vi "PlotCylDBparams.vi"() -> ()   [LabVIEW 2014]
uses:
  TypeDefs/RectHatch.ctl
  TypeDefs/PowerSpeed.ctl
  <vilib>/Utility/file.llb/Read From Spreadsheet File (DBL).vi
panel:
  in  "CircHatch":T1={"Diameter"=1.6, "Angle"=45.0, "Offset"=0.05, "Spacing"=0.1} {"Spacing" format="%#_13g"; "Offset" format="%#_13g"; "Diameter" format="%#_13g"}
  out "Params":cluster{dbl, dbl, dbl, dbl}[](array[cluster])=[{-5.0, 14.0, 382.0, 300.0}, {-5.0, 10.0, 370.0, 300.0}, {-5.0, 6.0, 360.0, 300.0}, {-5.0, 2.0, 350.0, 300.0}, {-5.0, -2.0, 340.0, 300.0}, {-5.0, -6.0, 330.0, 300.0}, {-5.0, -10.0, 320.0, 300.0}, {-5.0, -14.0, 310.0, 300.0}]
  in  "DummyCubeLoc":cluster{dbl, dbl}={-30.0, 30.0}
  in  "Save?":bool=TRUE
  in  "Path":path=path "\\\\nif-prgms-srvr.llnl.gov\\LMOT/Damage Group/Matthews/AM/fraunhofer SLM/BuildFiles_STL_ILT/SCN/DogBoneAndCylinders_11-23-16"
  in  "HighPower":dbl=300.0
  in  "Display":T2={"Mode"=enum."Inherit Value", "PointSize"=1.0, "LineWidth"=1.0}
  in  "LayerEnd":u32=266
  in  "LayerStart":u32
  in  "HatchPow":T3={"Power"=350.0, "Mark Speed"=300.0, "Jump Speed"=1000.0}
  in  "RectHatch":T4={"Width"=10.0, "Height"=1.0, "Angle"=45.0, "OffX"=0.1, "OffY"=0.1, "Spacing"=0.1} {"Spacing" format="%#_13g"; "OffY" format="%#_13g"; "OffX" format="%#_13g"; "Height" format="%#_13g"; "Width" format="%#_13g"}
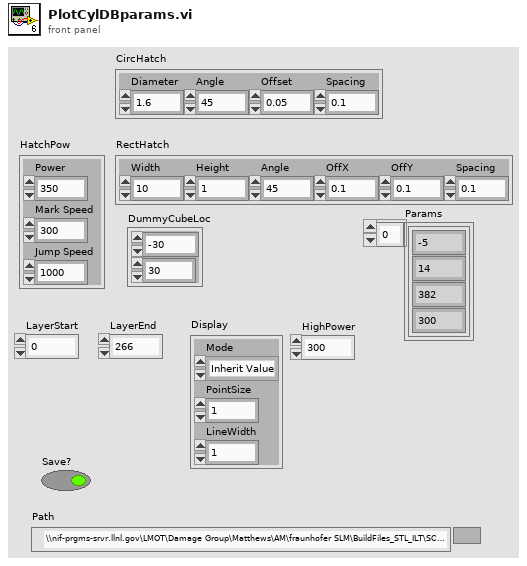
[diagram p1: front panel]
types:
  T1 = cluster{"Diameter":dbl, "Angle":sgl, "Offset":dbl, "Spacing":dbl}
  T2 = cluster{"Mode":enum16{"Inherit Value", "Points", "Wireframe", "Polygons"}, "PointSize":sgl, "LineWidth":sgl}
  T3 = typedef "PowerSpeed.ctl" = cluster{"Power":dbl, "Mark Speed":dbl, "Jump Speed":dbl}
  T4 = typedef "RectHatch.ctl" = cluster{"Width":dbl, "Height":dbl, "Angle":sgl, "OffX":dbl, "OffY":dbl, "Spacing":dbl}
  T5 = typedef "PathSupreme.ctl" = cluster{"VelocityProfiles":T6[], "Path":T7}
  T6 = typedef "VelocityProfile.ctl" = cluster{"ID":u32, "Velocity":dbl, "Mode":string, "tV1":u32, "tV2":u32, "tL1":u32, "tL2":u32}
  T7 = typedef "PathCut.ctl" = cluster{"Type":string, "Tag":string, "Segments":T8[]}
  T8 = typedef "Segment.ctl" = cluster{"SegmentID":u16, "Power":sgl, "idxVelocityProfile":u16, "End":cluster{"X":sgl, "Y":sgl}}
  T9 = typedef "Point3D.ctl" = cluster{"X":sgl, "Y":sgl, "Z":sgl}
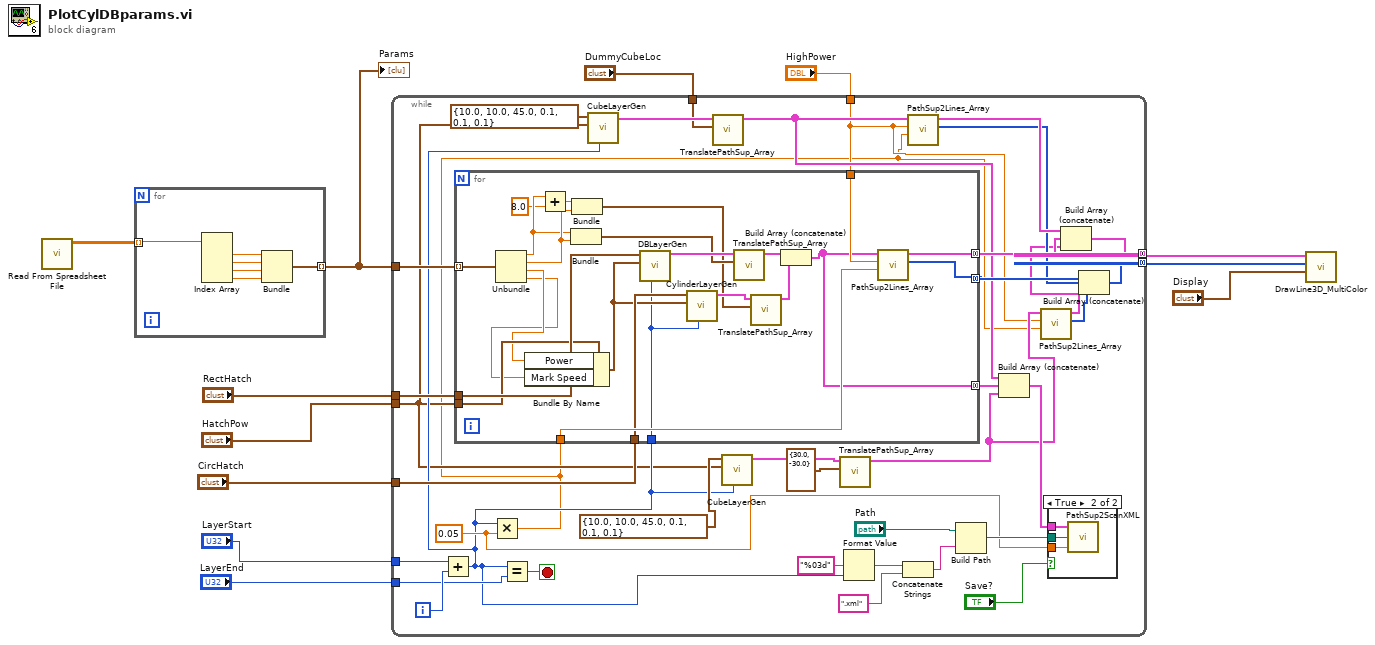
[diagram p0: block diagram]
diagram:
  n1 = call-poly <vilib>:"Read From Spreadsheet File.vi"() -> ("all rows"=w12:dbl[][])  [unwired: 7 in, 4 out]
  n2 = for {
    tunnel: w12 -> [w18] mode=indexing
    tunnel: [w13] -> w7 mode=indexing
    n3 = Index Array(array=w18) -> (element #1=w16:dbl, element #2=w17:dbl, element #3=w15:dbl, element #4=w14:dbl)  [unwired: 4 in]
    n4 = Bundle(w16, w17, w15, w14) -> (w13:cluster{dbl, dbl, dbl, dbl})  [unwired: 1 in]
  }
  "Params" <- w7
  n5 = while {
    tunnel: "HighPower" -> [w22]
    tunnel: [w38] -> w10 mode=concatenating
    tunnel: [w35] -> w9 mode=concatenating
    tunnel: w7 -> [w53]
    tunnel: "RectHatch" -> [w31]
    tunnel: "HatchPow" -> [w26]
    tunnel: "LayerEnd" -> [w52]
    tunnel: "LayerStart" -> [w51]
    tunnel: "DummyCubeLoc" -> [w41]
    tunnel: "CircHatch" -> [w30]
    i -> [w55]
    stop <- w54 stop-if-true
    w44 = 0.05 ("y")
    n6 = Add(x=w51, y=w55) -> (x+y=w27:u32)
    n7 = Multiply(x=w27, y=w44) -> (x*y=w21:dbl)
    n8 = for {
      tunnel: w27 -> [w68]
      tunnel: w21 -> [w78]
      tunnel: w22 -> [w75]
      tunnel: [w81] -> w39 mode=concatenating
      tunnel: w53 -> [w80] mode=indexing
      tunnel: w31 -> [w79]
      tunnel: w26 -> [w73]
      tunnel: [w59] -> w34 mode=concatenating
      tunnel: [w74] -> w37 mode=concatenating
      tunnel: w30 -> [w70]
      n9 = Unbundle(w80) -> (w64:dbl, w66:dbl, w72:dbl, w71:dbl)
      n10 = Bundle By Name(cluster=w73, "Power"=w72, "Mark Speed"=w71) -> (w69:T3)
      n11 = Add(x=w64, y=8.0) -> (x+y=w65:dbl)
      n12 = Bundle(w64, w66) -> (w76:cluster{dbl, dbl})  [unwired: 1 in]
      n13 = Bundle(w65, w66) -> (w61:cluster{dbl, dbl})  [unwired: 1 in]
      n14 = call "DBLayerGen.vi"("Layer"=w68, "HatchPow"=w69, "RectHatch"=w79) -> ("PathSups"=w77:T5[])  [unwired: 8 in]
      n15 = call "CylinderLayerGen.vi"("Layer"=w68, "HatchPow"=w69, "CircHatch"=w70) -> ("PathSups"=w62:T5[])  [unwired: 8 in]
      n16 = call "TranslatePathSup_Array.vi"("Offset"=w76, "PathSupsIn"=w77) -> ("PathSupsOut"=w67:T5[])  [unwired: 9 in]
      n17 = call "TranslatePathSup_Array.vi"("Offset"=w61, "PathSupsIn"=w62) -> ("PathSupsOut"=w60:T5[])  [unwired: 9 in]
      n18 = Build Array (concatenate)(w67, w60) -> (w59:T5[])
      n19 = call "PathSup2Lines_Array.vi"("Z"=w78, "HighPower"=w75, "PathSupIn"=w59) -> ("Colors"=w74:u32[], "Lines"=w81:cluster{"P0":T9, "P1":T9}[])  [unwired: 7 in]
    }
    n20 = Equal?(x=w27, y=w52) -> (x = y?=w54:bool)
    n21 = call "CubeLayerGen.vi"("Layer"=w27, "HatchPow"=w26, "RectHatch"=T4 {"Width"=10.0, "Height"=10.0, "Angle"=45.0, "OffX"=0.1, "OffY"=0.1, "Spacing"=0.1}) -> ("PathSups"=w42:T5[])  [unwired: 8 in]
    n22 = call "TranslatePathSup_Array.vi"("Offset"=w41, "PathSupsIn"=w42) -> ("PathSupsOut"=w33:T5[])  [unwired: 9 in]
    n23 = call "CubeLayerGen.vi"("Layer"=w27, "HatchPow"=w26, "RectHatch"=T4 {"Width"=10.0, "Height"=10.0, "Angle"=45.0, "OffX"=0.1, "OffY"=0.1, "Spacing"=0.1}) -> ("PathSups"=w25:T5[])  [unwired: 8 in]
    n24 = call "TranslatePathSup_Array.vi"("Offset"=cluster{dbl, dbl} {30.0, -30.0}, "PathSupsIn"=w25) -> ("PathSupsOut"=w23:T5[])  [unwired: 9 in]
    n25 = Format Value(format string="%03d", value (0)=w27) -> (output string=w49:string)  [unwired: 1 in]
    n26 = Concatenate Strings(w49, ".xml" ("string")) -> (w47:string)
    n27 = call "PathSup2Lines_Array.vi"("Z"=w21, "HighPower"=w22, "PathSupIn"=w33) -> ("Colors"=w36:u32[], "Lines"=w40:cluster{"P0":T9, "P1":T9}[])  [unwired: 7 in]
    n28 = Build Path(base path="Path", name or relative path=w47) -> (appended path=w45:path)
    n29 = Build Array (concatenate)(w33, w34, w23) -> (w32:T5[])
    n30 = call "PathSup2Lines_Array.vi"("Z"=w21, "HighPower"=w22, "PathSupIn"=w23) -> ("Colors"=w19:u32[], "Lines"=w20:cluster{"P0":T9, "P1":T9}[])  [unwired: 7 in]
    n31 = case shown="True" "Save?" {
      tunnel: w32 -> [_ w58]
      tunnel: w45 -> [_ w57]
      tunnel: w44 -> [_ w56]
      frame False {
      }
      frame True {
        n32 = call "PathSup2ScanXML.vi"("Thickness"=w56, "Path"=w57, "PathSupremes"=w58) -> ()  [unwired: 2 in, 1 out]
      }
    }
    n33 = Build Array (concatenate)(w40, w39, w20) -> (w38:cluster{"P0":T9, "P1":T9}[])
    n34 = Build Array (concatenate)(w37, w36, w19) -> (w35:u32[])
  }
  n35 = call "DrawLine3D_MultiColor.vi"("Display"="Display", "Colors"=w9, "Lines"=w10) -> ()  [unwired: 9 in]
